vi "SeCrTs-DO Data FGV.vi"(0 "DO Values In":bool[](array[boolean]), 1 "Option":T1(ring)=enum."Start Pattern Mode", 5 "DO Channel Names":string[](array[string]), 7 "initiate":bool, 9 "Time Stamp In":timestamp, 11 "error in (no error)":errorcluster, 12 "DO Pattern Values In":bool[][](array[boolean])) -> (3 "Expected Completed Time (Pattern)":timestamp, 4 "DO Values Out":bool[](array[boolean]), 6 "All data out":waveform(dbl)[](array[waveform]), 8 "DO Channel Names Out":string[](array[string]), 10 "DO Waveform Out":digitalwaveform[](array[waveform]), 14 "Time Stamp Out":timestamp, 15 "error out":errorcluster)   [LabVIEW 2022 SP3]
uses:
  RT Controls/SeCrTs-FGV Read write.ctl
  <vilib>/Waveform/DTblOps.llb/DTbl Boolean Array to Digital.vi
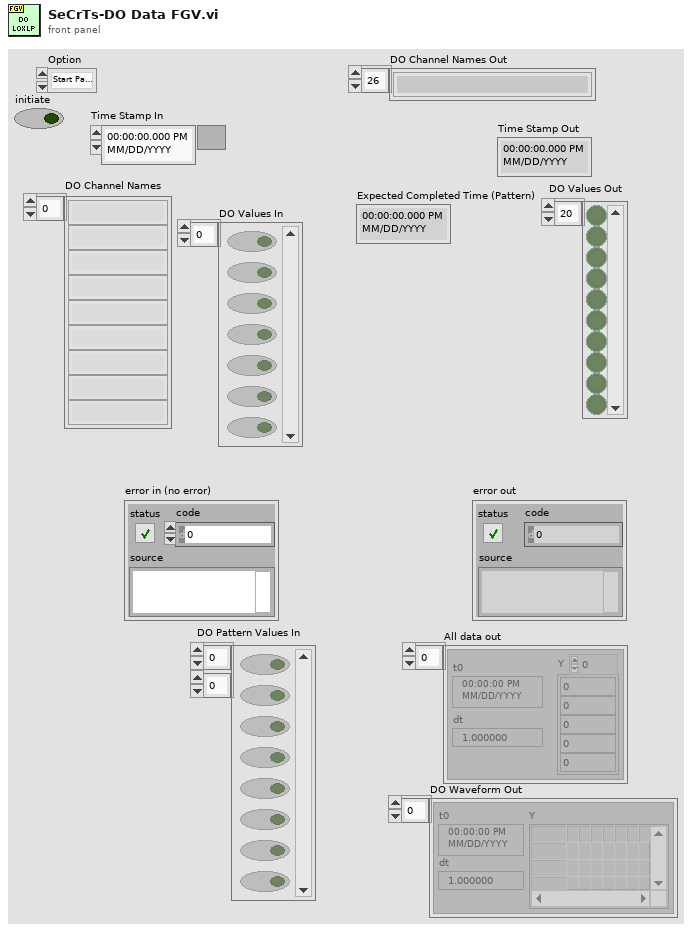
[diagram p1: front panel]
types:
  T1 = enum16{"Init", "Read", "Write 'All'", "Write 'n'", "Write Safe Value", "Write Start Time", "Overwrite Pattern", "Overwrite Pattern with Start", "Append Pattern", "Start Pattern Mode", "Abort Pattern Mode", "Read 1"}
  T2 = typedef "SeCrTs-FGV Read write.ctl" = enum16{"Write", "Read"}
  T3 = cluster{"Samples to Read":i32, "Pattern Mode?":bool, "dt(sec)":dbl, "DO Init Time (Samples)":i32, "dt per Read/Write":dbl, "Write Pointer":i32, "Pattern Size":i32, "Loop Rate (mSec)":i32, "Buffer Size (Samples)":i32, "Sampling rate":dbl, "Max DO Delay Time (samples)":dbl, "Min DO Delay Time (samples)":dbl, "Queue Size":i32, "DO Init Sample Duration (Sec)":dbl}
  T4 = cluster{"Pattern Size":i32, "Write Pointer":i32, "DO Channel Names":string[], "Pattern Mode?":bool, "DO Safe Waveform":waveform(dbl)[], "DO Safe Digital Waveform":digitalwaveform[], "DO Safe Values In":bool[], "dt per Read/Write":dbl}
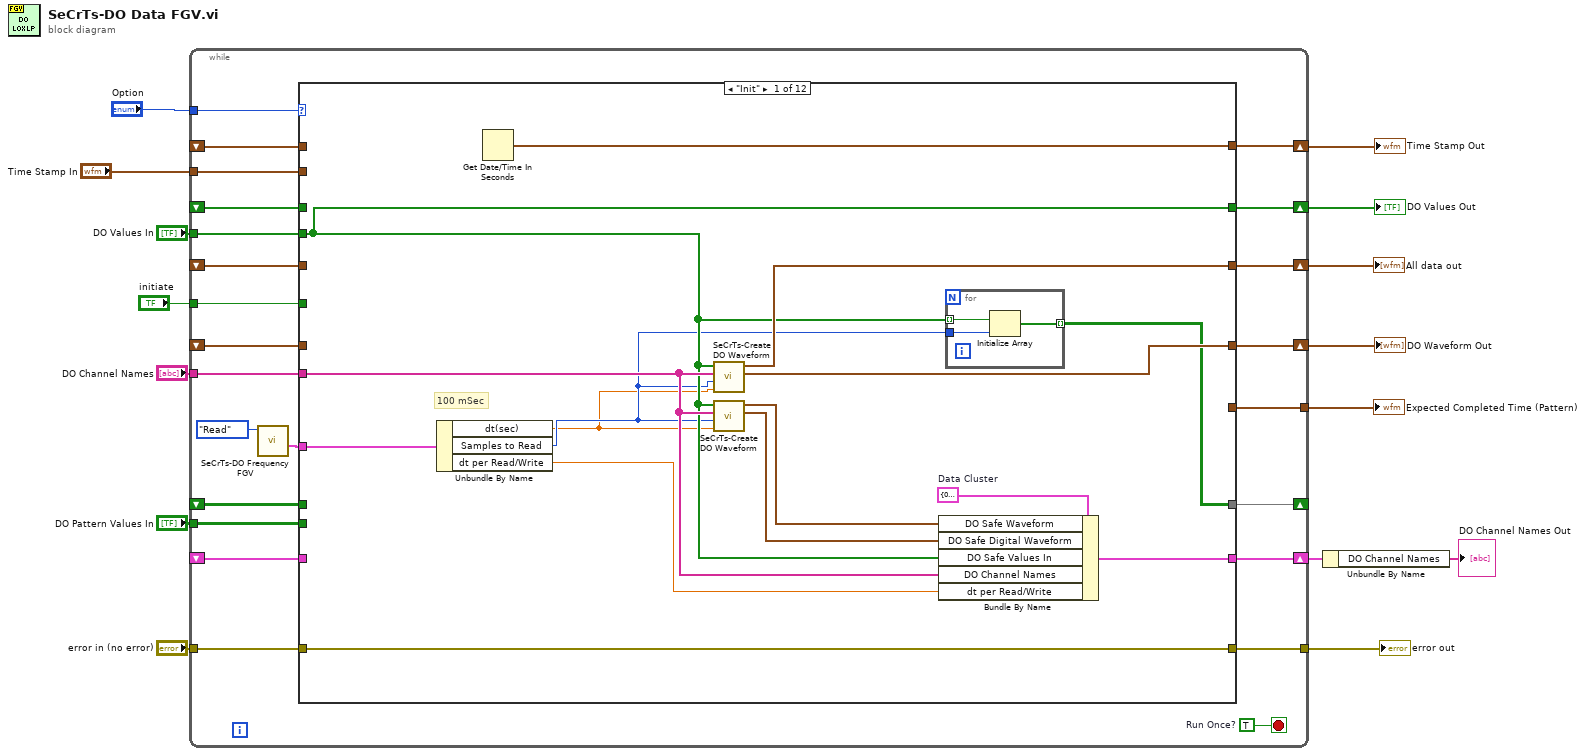
[diagram p0: block diagram]
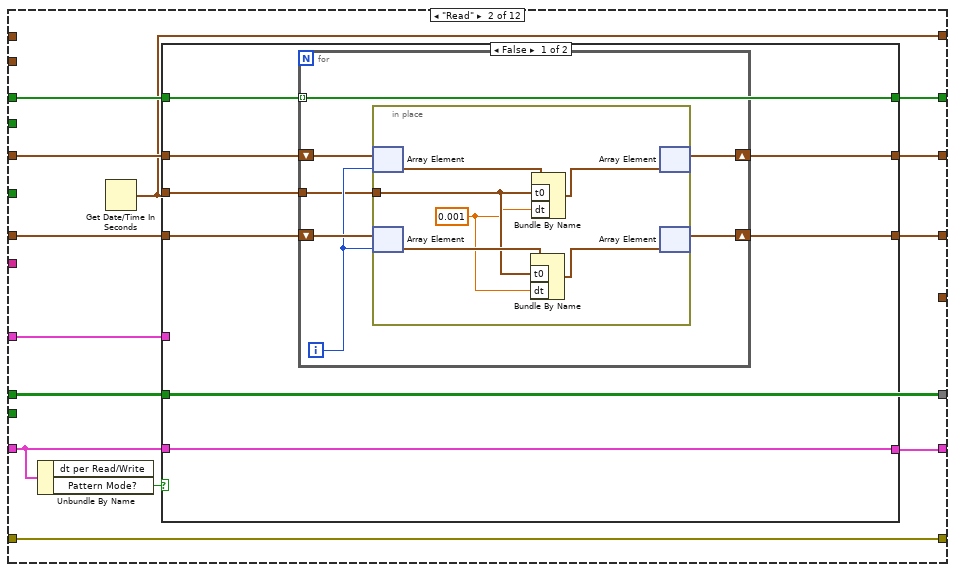
[diagram p2: hidden frame]
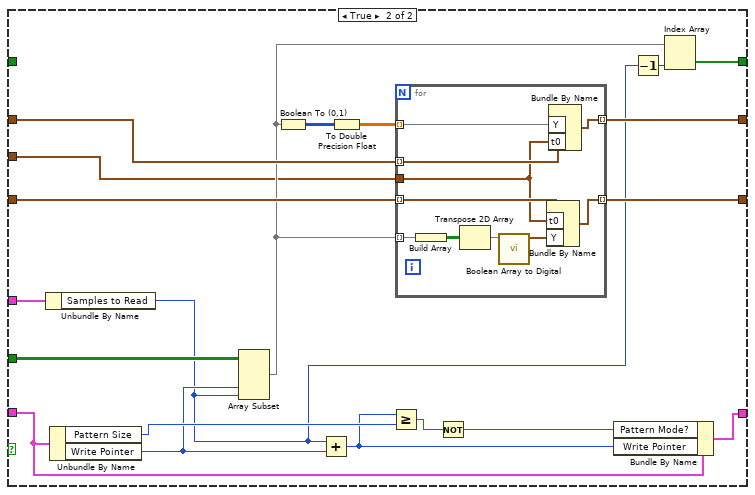
[diagram p3: hidden frame]
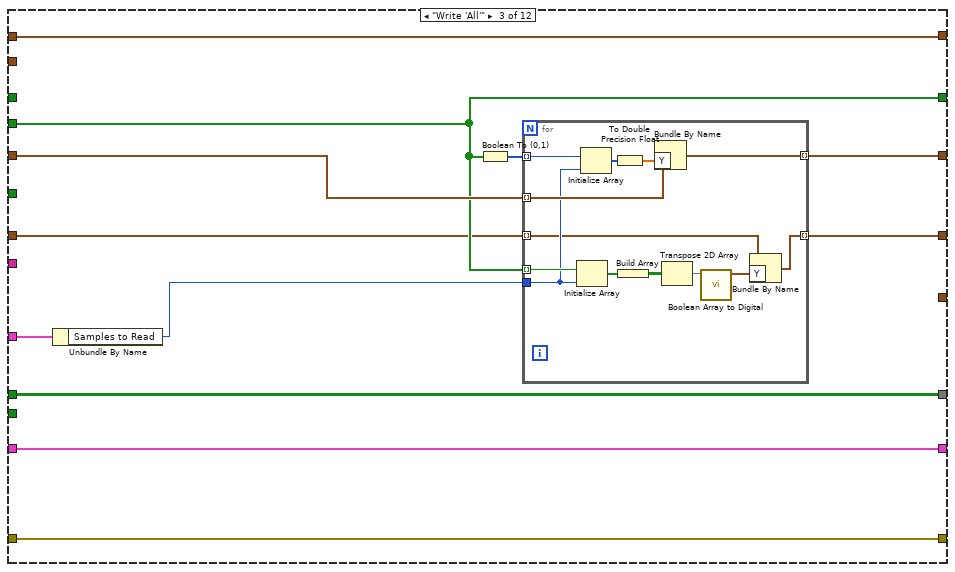
[diagram p4: hidden frame]
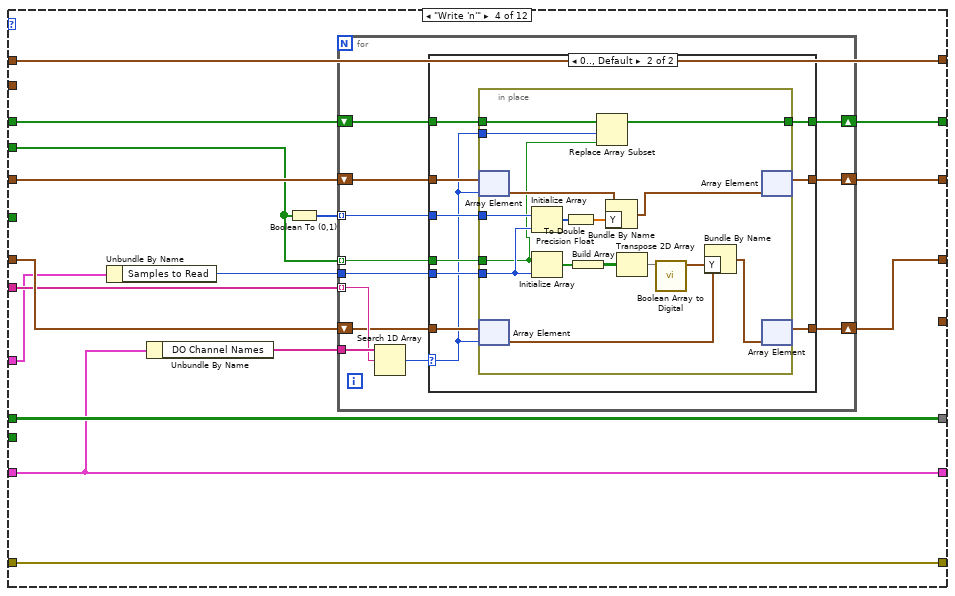
[diagram p5: hidden frame]
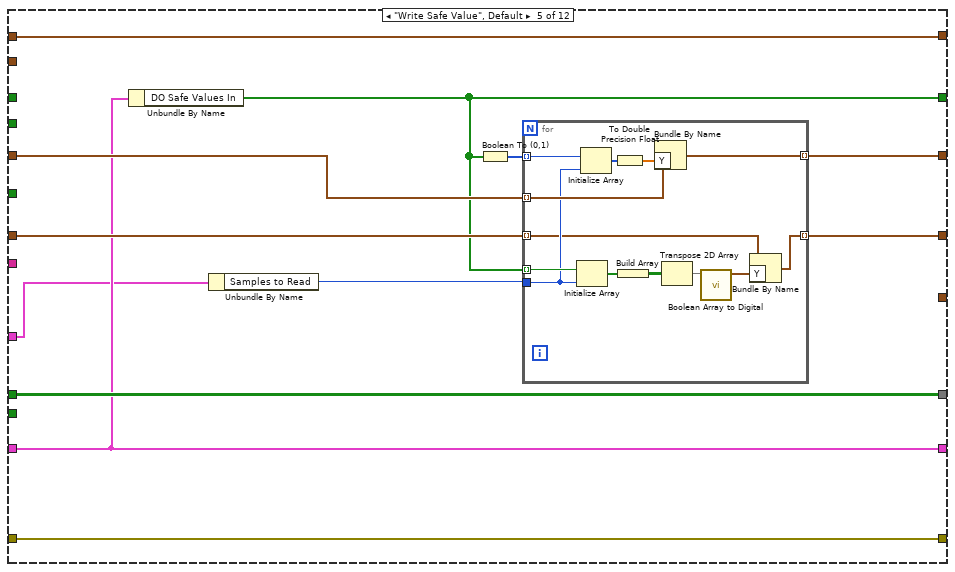
[diagram p7: hidden frame]
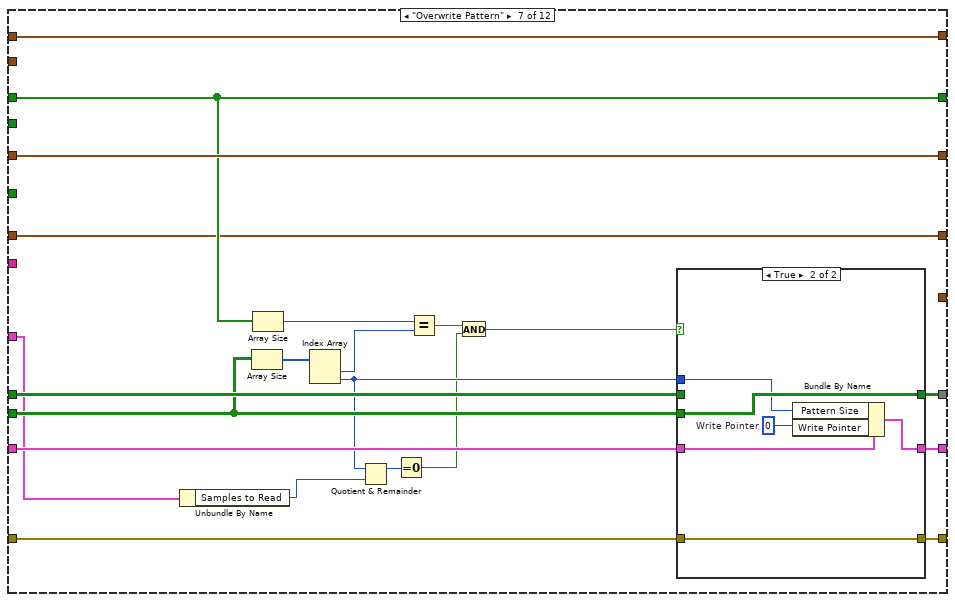
[diagram p9: hidden frame]
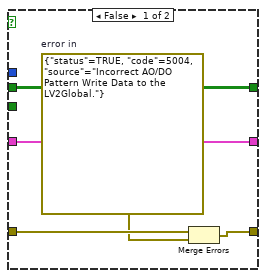
[diagram p10: hidden frame]
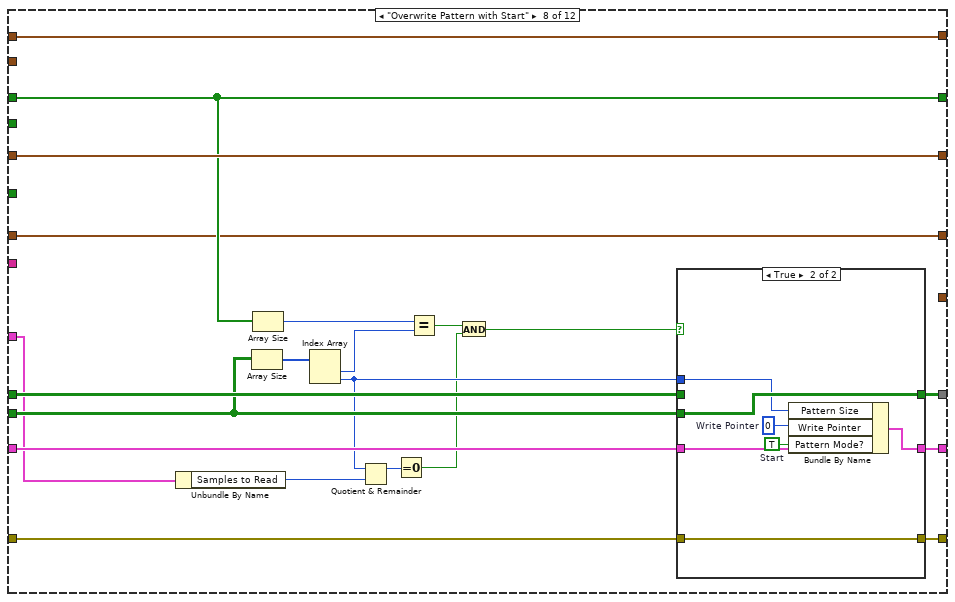
[diagram p11: hidden frame]
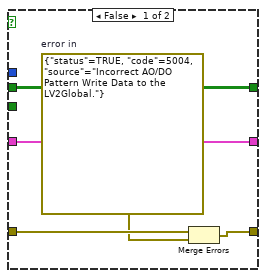
[diagram p12: hidden frame]
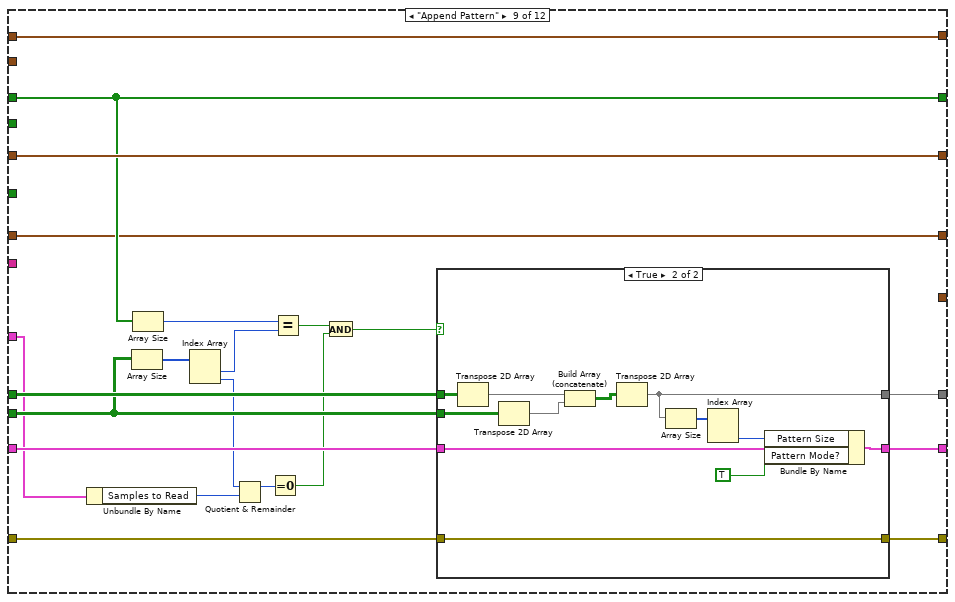
[diagram p13: hidden frame]
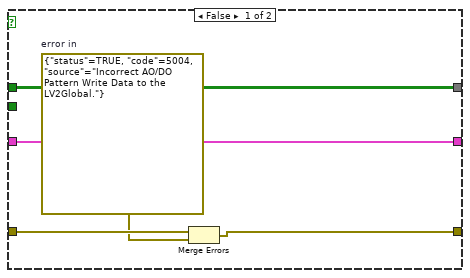
[diagram p14: hidden frame]
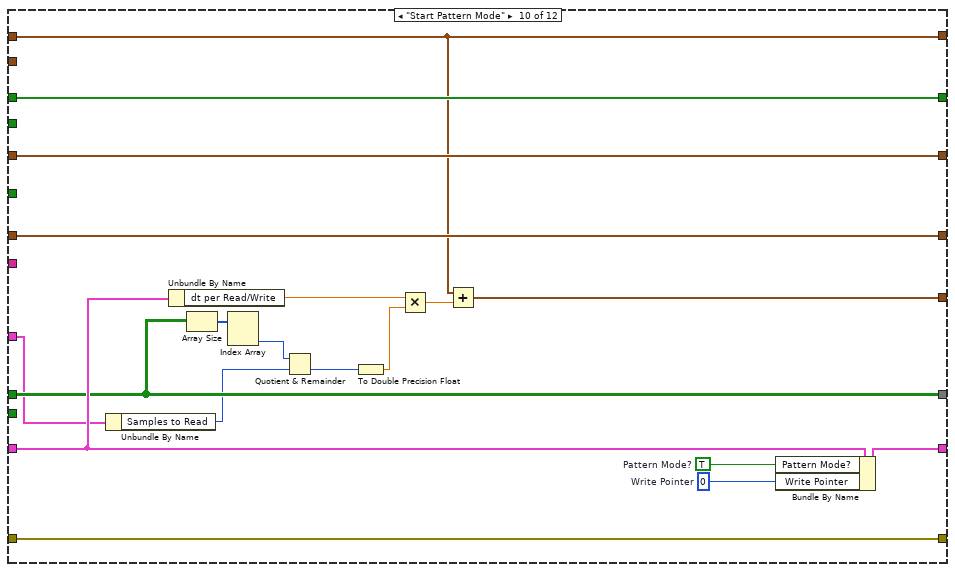
[diagram p15: hidden frame]
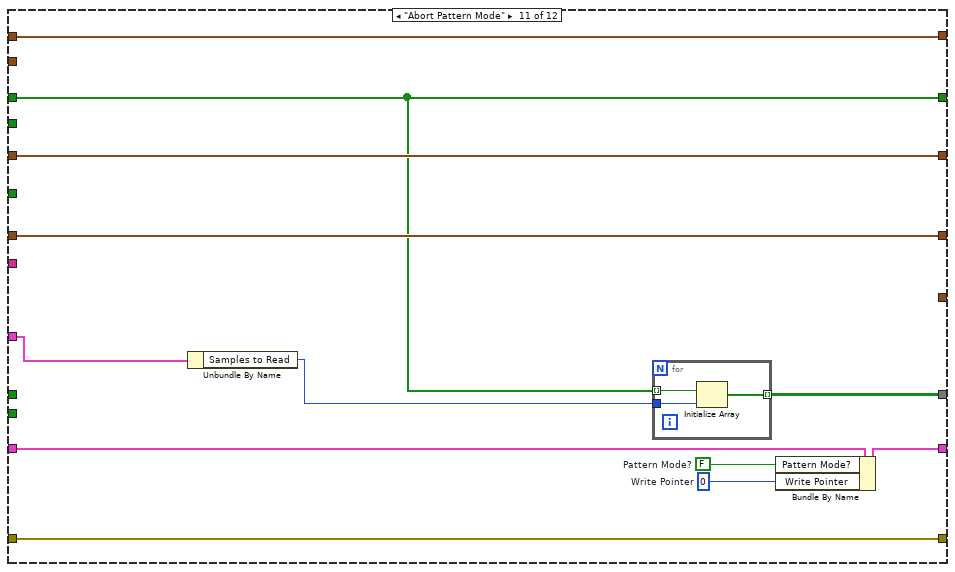
[diagram p16: hidden frame]
diagram:
  n1 = while {
    tunnel: "DO Values In" -> [w37]
    shift-right: [w38] -> w15
    shift-left: _ -> [w36]
    shift-right: [w35] -> w13
    shift-left: _ -> [w34]
    shift-right: [w33] -> w12
    shift-left: _ -> [w32]
    tunnel: "DO Pattern Values In" -> [w29]
    shift-right: [w30] -> _
    shift-left: _ -> [w28]
    shift-right: [w27] -> w3
    shift-left: _ -> [w26]
    tunnel: "error in (no error)" -> [w25]
    tunnel: [w24] -> w8
    tunnel: "DO Channel Names" -> [w23]
    shift-right: [w31] -> w11
    shift-left: _ -> [w22]
    tunnel: "Time Stamp In" -> [w21]
    tunnel: [w20] -> w5
    tunnel: "Option" -> [w19]
    tunnel: "initiate" -> [w17]
    stop <- w39 stop-if-true
    w39 = TRUE  # Run Once?
    n2 = call "SeCrTs-DO Frequency  FGV.vi"("Write/Read"=SeCrTs-FGV_Read_write."Read") -> ("DO Set Frequency (R)"=w18:T3)  [unwired: 9 in, 1 out]
    n3 = case shown="\"Init\"" w19 {
      tunnel: [w45 w61 w126 w147 w204 w233 w252 w284 w317 w355 w360 w377] -> w38
      tunnel: w37 -> [w45 _ w126 w156 _ _ _ _ _ _ _ _]
      tunnel: w36 -> [_ w66 _ w148 _ w233 w252 w284 w317 w355 w360 w377]
      tunnel: [w54 w58 w131 w160 w213 w227 w254 w286 w319 w347 w367 w371] -> w35
      tunnel: w34 -> [_ _ w131 w160 w213 _ w254 w286 w319 w347 w367 w371]
      tunnel: [w50 w62 w124 w154 w208 w232 w253 w285 w318 w354 w366 w372] -> w33
      tunnel: w32 -> [_ w67 w127 w157 w210 w232 w253 w285 w318 w354 w366 w372]
      tunnel: [w49 w63 w123 w153 w207 w231 w238 w270 w301 w353 w365 w373] -> w31
      tunnel: [w44 w60 w130 w159 w212 w230 w246 w278 w310 w346 w359 w376] -> w30
      tunnel: w29 -> [_ _ _ _ _ _ w244 w276 w308 _ _ _]
      tunnel: w28 -> [_ w60 w130 w159 w212 w230 w245 w277 w309 w346 _ w376]
      tunnel: [w51 w64 w129 w150 w205 w229 w247 w279 w312 w351 w362 w375] -> w27
      tunnel: w26 -> [_ w65 w129 w150 w205 w229 w248 w280 w313 w348 w364 w375]
      tunnel: w25 -> [w52 w70 w128 w158 w211 w228 w243 w275 w307 w352 w363 w374]
      tunnel: [w52 w70 w128 w158 w211 w228 w242 w274 w306 w352 w363 w374] -> w24
      tunnel: w23 -> [w48 _ _ w151 _ _ _ _ _ _ _ _]
      tunnel: w22 -> [_ w68 w122 w152 w206 w231 w238 w270 w301 w353 w365 w373]
      tunnel: w21 -> [_ _ _ _ _ w227 _ _ _ _ _ _]
      tunnel: [_ _ _ _ _ _ _ _ _ w340 _ _] -> w20
      tunnel: w18 -> [w43 w59 w121 w146 w202 _ w234 w266 w300 w337 w356 _]
      tunnel: w17 -> [_ _ _ _ _ _ _ _ _ _ _ _]
      frame "Init" {
        w53 = T4 {"Pattern Size"=0, "Write Pointer"=0, "DO Channel Names"=[], "Pattern Mode?"=FALSE, "DO Safe Waveform"=[], "DO Safe Digital Waveform"=[], "DO Safe Values In"=[], "dt per Read/Write"=100.0}  # Data Cluster
        # "100 mSec"
        n4 = Unbundle By Name(w43) -> ("dt(sec)"=w41:dbl, "Samples to Read"=w42:i32, "dt per Read/Write"=w40:dbl)
        n5 = Get Date/Time In Seconds() -> (seconds since 1Jan1904=w54:timestamp)
        n6 = call "SeCrTs-Create DO Waveform.vi"("dt(sec)"=w41, "Size"=w42, "DO Channel Names"=w48, "DO Values In"=w45) -> ("DO Digital Waveform"=w49:digitalwaveform[], "DO Waveform"=w50:waveform(dbl)[])  [unwired: 6 in]
        n7 = call "SeCrTs-Create DO Waveform.vi"("dt(sec)"=w41, "Size"=w42, "DO Channel Names"=w48, "DO Values In"=w45) -> ("DO Digital Waveform"=w46:digitalwaveform[], "DO Waveform"=w47:waveform(dbl)[])  [unwired: 6 in]
        n8 = Bundle By Name(cluster=w53, "DO Safe Waveform"=w47, "DO Safe Digital Waveform"=w46, "DO Safe Values In"=w45, "DO Channel Names"=w48, "dt per Read/Write"=w40) -> (w51:T4)
        n9 = for {
          tunnel: w42 -> [w57]
          tunnel: w45 -> [w56] mode=indexing
          tunnel: [w55] -> w44 mode=indexing
          n10 = Initialize Array(w56, w57) -> (w55:bool[])
        }
      }
      frame "Read" {
        n11 = Unbundle By Name(w65) -> ("Pattern Mode?"=w69:bool)  [unwired: 1 out]
        n12 = Get Date/Time In Seconds() -> (seconds since 1Jan1904=w58:timestamp)
        n13 = case shown="False" w69 {
          tunnel: w60 -> [_ w107]
          tunnel: w68 -> [w75 w106]
          tunnel: w67 -> [w76 w103]
          tunnel: w66 -> [w71 _]
          tunnel: w65 -> [w77 w109]
          tunnel: [w77 w108] -> w64
          tunnel: [w73 w105] -> w63
          tunnel: [w74 w104] -> w62
          tunnel: [w71 w101] -> w61
          tunnel: w58 -> [w72 w95]
          tunnel: w59 -> [_ w91]
          frame False {
            n14 = for {
              shift-right: [w80] -> w74
              shift-left: w76 -> [w83]
              shift-right: [w81] -> w73
              shift-left: w75 -> [w82]
              tunnel: w72 -> [w78]
              tunnel: w71 -> [_] mode=indexing
              i -> [w79]
              n15 = in-place {
                in-place-border: w78 -> [w85]
                w84 = 0.001 ("dt")
                n16 = in-place-array #1(w83, w79) -> (w89:waveform(dbl))
                n17 = in-place-array #2(w82, w79) -> (w87:digitalwaveform)
                n18 = Bundle By Name(cluster=w87, "t0"=w85, "dt"=w84) -> (w86:digitalwaveform)
                n19 = Bundle By Name(cluster=w89, "t0"=w85, "dt"=w84) -> (w88:waveform(dbl))
                n20 = in-place-array #1(w88) -> (w80:waveform(dbl)[])  [unwired: 1 out]
                n21 = in-place-array #2(w86) -> (w81:digitalwaveform[])  [unwired: 1 out]
              }
            }
          }
          frame True {
            n22 = Unbundle By Name(w91) -> ("Samples to Read"=w90:i32)
            n23 = Unbundle By Name(w109) -> ("Pattern Size"=w99:i32, "Write Pointer"=w94:i32)
            n24 = Array Subset(array=w107, index (col)=w94, length (col)=w90) -> (w102:bool[][])  [unwired: 2 in]
            n25 = Boolean To (0,1)(Boolean=w102) -> (0, 1=w97:i16[][])
            n26 = Add(x=w90, y=w94) -> (x+y=w93:i32)
            n27 = To Double Precision Float(number=w97) -> (double precision float=w96:dbl[][])
            n28 = Greater Or Equal?(x=w93, y=w99) -> (x >= y?=w98:bool)
            n29 = for {
              tunnel: [w119] -> w104 mode=indexing
              tunnel: w103 -> [w118] mode=indexing
              tunnel: w102 -> [w112] mode=indexing
              tunnel: [w115] -> w105 mode=indexing
              tunnel: w106 -> [w113] mode=indexing
              tunnel: w96 -> [w111] mode=indexing
              tunnel: w95 -> [w110]
              n30 = Build Array(w112) -> (w117:bool[][])
              n31 = Transpose 2D Array(2D array=w117) -> (transposed array=w114:bool[][])
              n32 = call-poly <vilib>:"Boolean Array to Digital.vi"("boolean array"=w114) -> ("digital data"=w116:digitaldata)  [unwired: 9 in, 1 out]
              n33 = Bundle By Name(cluster=w113, "t0"=w110, "Y"=w116) -> (w115:digitalwaveform)
              n34 = Bundle By Name(cluster=w118, "Y"=w111, "t0"=w110) -> (w119:waveform(dbl))
            }
            n35 = Not(x=w98) -> (.not. x?=w92:bool)
            n36 = Bundle By Name(cluster=w109, "Pattern Mode?"=w92, "Write Pointer"=w93) -> (w108:T4)
            n37 = Decrement(x=w90) -> (x-1=w100:i32)
            n38 = Index Array(array=w102, index (col)=w100) -> (element=w101:bool[])  [unwired: 1 in]
          }
        }
      }
      frame "Write 'All'" {
        n39 = Unbundle By Name(w121) -> ("Samples to Read"=w120:i32)
        n40 = Boolean To (0,1)(Boolean=w126) -> (0, 1=w125:i16[])
        n41 = for {
          tunnel: w125 -> [w143] mode=indexing
          tunnel: [w144] -> w124 mode=indexing
          tunnel: w120 -> [w138]
          tunnel: w127 -> [w140] mode=indexing
          tunnel: w126 -> [w139] mode=indexing
          tunnel: [w134] -> w123 mode=indexing
          tunnel: w122 -> [w132] mode=indexing
          n42 = Initialize Array(w139, w138) -> (w137:bool[])
          n43 = Initialize Array(w143, w138) -> (w142:i16[])
          n44 = To Double Precision Float(number=w142) -> (double precision float=w141:dbl[])
          n45 = Build Array(w137) -> (w136:bool[][])
          n46 = Bundle By Name(cluster=w140, "Y"=w141) -> (w144:waveform(dbl))
          n47 = Transpose 2D Array(2D array=w136) -> (transposed array=w133:bool[][])
          n48 = call-poly <vilib>:"Boolean Array to Digital.vi"("boolean array"=w133) -> ("digital data"=w135:digitaldata)  [unwired: 9 in, 1 out]
          n49 = Bundle By Name(cluster=w132, "Y"=w135) -> (w134:digitalwaveform)
        }
      }
      frame "Write 'n'" {
        n50 = Unbundle By Name(w146) -> ("Samples to Read"=w145:i32)
        n51 = Unbundle By Name(w150) -> ("DO Channel Names"=w149:string[])
        n52 = Boolean To (0,1)(Boolean=w156) -> (0, 1=w155:i16[])
        n53 = for {
          tunnel: w155 -> [w171] mode=indexing
          tunnel: w145 -> [w169]
          tunnel: w156 -> [w170] mode=indexing
          shift-right: [w163] -> w153
          shift-left: w152 -> [w165]
          tunnel: w151 -> [w167] mode=indexing
          tunnel: w149 -> [w168]
          shift-right: [w172] -> w154
          shift-left: w157 -> [w164]
          shift-right: [w161] -> w147
          shift-left: w148 -> [w162]
          n54 = Search 1D Array(1D array=w168, element=w167) -> (index of element=w166:i32)  [unwired: 1 in]
          n55 = case shown="0.., Default" w166 {
            selector: w166 -> [_ w176]
            tunnel: [w175 w180] -> w172
            tunnel: w171 -> [_ w185]
            tunnel: w170 -> [_ w184]
            tunnel: w169 -> [_ w183]
            tunnel: w165 -> [w174 w182]
            tunnel: w164 -> [w175 w181]
            tunnel: [w174 w179] -> w163
            tunnel: w162 -> [w173 w178]
            tunnel: [w173 w177] -> w161
            frame -1 {
            }
            frame 0.., Default {
              n56 = in-place {
                in-place-border: w185 -> [w201]
                in-place-border: w184 -> [w186]
                in-place-border: w183 -> [w198]
                in-place-border: w178 -> [w189]
                in-place-border: [w188] -> w177
                in-place-border: w176 -> [w187]
                n57 = in-place-array #3(w181, w176) -> (w191:waveform(dbl))
                n58 = in-place-array #4(w182, w176) -> (w193:digitalwaveform)
                n59 = Initialize Array(w201, w198) -> (w200:i16[])
                n60 = Initialize Array(w186, w198) -> (w197:bool[])
                n61 = To Double Precision Float(number=w200) -> (double precision float=w199:dbl[])
                n62 = Build Array(w197) -> (w196:bool[][])
                n63 = Replace Array Subset(array=w189, new element=w186, index=w187) -> (w188:bool[])
                n64 = Bundle By Name(cluster=w191, "Y"=w199) -> (w192:waveform(dbl))
                n65 = Transpose 2D Array(2D array=w196) -> (transposed array=w194:bool[][])
                n66 = call-poly <vilib>:"Boolean Array to Digital.vi"("boolean array"=w194) -> ("digital data"=w195:digitaldata)  [unwired: 9 in, 1 out]
                n67 = Bundle By Name(cluster=w193, "Y"=w195) -> (w190:digitalwaveform)
                n68 = in-place-array #3(w192) -> (w180:waveform(dbl)[])  [unwired: 1 out]
                n69 = in-place-array #4(w190) -> (w179:digitalwaveform[])  [unwired: 1 out]
              }
            }
          }
        }
      }
      frame "Write Safe Value", Default {
        n70 = Unbundle By Name(w205) -> ("DO Safe Values In"=w204:bool[])
        n71 = Unbundle By Name(w202) -> ("Samples to Read"=w203:i32)
        n72 = Boolean To (0,1)(Boolean=w204) -> (0, 1=w209:i16[])
        n73 = for {
          tunnel: w209 -> [w225] mode=indexing
          tunnel: [w226] -> w208 mode=indexing
          tunnel: w203 -> [w220]
          tunnel: w210 -> [w222] mode=indexing
          tunnel: w204 -> [w221] mode=indexing
          tunnel: [w216] -> w207 mode=indexing
          tunnel: w206 -> [w214] mode=indexing
          n74 = Initialize Array(w221, w220) -> (w219:bool[])
          n75 = Initialize Array(w225, w220) -> (w224:i16[])
          n76 = To Double Precision Float(number=w224) -> (double precision float=w223:dbl[])
          n77 = Build Array(w219) -> (w218:bool[][])
          n78 = Bundle By Name(cluster=w222, "Y"=w223) -> (w226:waveform(dbl))
          n79 = Transpose 2D Array(2D array=w218) -> (transposed array=w215:bool[][])
          n80 = call-poly <vilib>:"Boolean Array to Digital.vi"("boolean array"=w215) -> ("digital data"=w217:digitaldata)  [unwired: 9 in, 1 out]
          n81 = Bundle By Name(cluster=w214, "Y"=w217) -> (w216:digitalwaveform)
        }
      }
      frame "Write Start Time" {
      }
      frame "Overwrite Pattern" {
        n82 = Unbundle By Name(w234) -> ("Samples to Read"=w235:i32)
        n83 = Array Size(array=w244) -> (size(s)=w251:i32[])
        n84 = Array Size(array=w252) -> (size(s)=w249:i32)
        n85 = Index Array(array=w251) -> (element #1=w250:i32, element #2=w241:i32)  [unwired: 2 in]
        n86 = Quotient & Remainder(x=w241, y=w235) -> (x-y*floor(x/y)=w240:i32)  [unwired: 1 out]
        n87 = Equal To 0?(x=w240) -> (x = 0?=w236:bool)
        n88 = Equal?(x=w249, y=w250) -> (x = y?=w237:bool)
        n89 = And(x=w237, y=w236) -> (x .and. y?=w239:bool)
        n90 = case shown="True" w239 {
          tunnel: w248 -> [w259 w265]
          tunnel: [w259 w264] -> w247
          tunnel: w241 -> [_ w260]
          tunnel: [w258 w262] -> w246
          tunnel: w245 -> [w258 _]
          tunnel: w244 -> [_ w262]
          tunnel: w243 -> [w257 w261]
          tunnel: [w256 w261] -> w242
          frame False {
            w255 = errorcluster {"status"=TRUE, "code"=5004, "source"="Incorrect AO/DO Pattern Write Data to the LV2Global."}  # error in
            n91 = Merge Errors(w257, w255) -> (w256:errorcluster)
          }
          frame True {
            w263 = 0  # Write Pointer
            n92 = Bundle By Name(cluster=w265, "Pattern Size"=w260, "Write Pointer"=w263) -> (w264:T4)
          }
        }
      }
      frame "Overwrite Pattern with Start" {
        n93 = Unbundle By Name(w266) -> ("Samples to Read"=w267:i32)
        n94 = Array Size(array=w276) -> (size(s)=w283:i32[])
        n95 = Array Size(array=w284) -> (size(s)=w281:i32)
        n96 = Index Array(array=w283) -> (element #1=w282:i32, element #2=w273:i32)  [unwired: 2 in]
        n97 = Quotient & Remainder(x=w273, y=w267) -> (x-y*floor(x/y)=w272:i32)  [unwired: 1 out]
        n98 = Equal To 0?(x=w272) -> (x = 0?=w268:bool)
        n99 = Equal?(x=w281, y=w282) -> (x = y?=w269:bool)
        n100 = And(x=w269, y=w268) -> (x .and. y?=w271:bool)
        n101 = case shown="True" w271 {
          tunnel: w280 -> [w291 w298]
          tunnel: [w291 w297] -> w279
          tunnel: w273 -> [_ w292]
          tunnel: [w290 w295] -> w278
          tunnel: w277 -> [w290 _]
          tunnel: w276 -> [_ w295]
          tunnel: w275 -> [w289 w294]
          tunnel: [w288 w294] -> w274
          frame False {
            w287 = errorcluster {"status"=TRUE, "code"=5004, "source"="Incorrect AO/DO Pattern Write Data to the LV2Global."}  # error in
            n102 = Merge Errors(w289, w287) -> (w288:errorcluster)
          }
          frame True {
            w293 = TRUE  # Start
            w296 = 0  # Write Pointer
            n103 = Bundle By Name(cluster=w298, "Pattern Size"=w292, "Write Pointer"=w296, "Pattern Mode?"=w293) -> (w297:T4)
          }
        }
      }
      frame "Append Pattern" {
        n104 = Unbundle By Name(w300) -> ("Samples to Read"=w299:i32)
        n105 = Array Size(array=w308) -> (size(s)=w316:i32[])
        n106 = Array Size(array=w317) -> (size(s)=w314:i32)
        n107 = Index Array(array=w316) -> (element #1=w315:i32, element #2=w304:i32)  [unwired: 2 in]
        n108 = Quotient & Remainder(x=w304, y=w299) -> (x-y*floor(x/y)=w305:i32)  [unwired: 1 out]
        n109 = Equal To 0?(x=w305) -> (x = 0?=w302:bool)
        n110 = Equal?(x=w314, y=w315) -> (x = y?=w311:bool)
        n111 = And(x=w311, y=w302) -> (x .and. y?=w303:bool)
        n112 = case shown="True" w303 {
          tunnel: w313 -> [w324 w336]
          tunnel: [w324 w335] -> w312
          tunnel: [w323 w327] -> w310
          tunnel: w309 -> [w323 w333]
          tunnel: w308 -> [_ w332]
          tunnel: w307 -> [w322 w334]
          tunnel: [w321 w334] -> w306
          frame False {
            w320 = errorcluster {"status"=TRUE, "code"=5004, "source"="Incorrect AO/DO Pattern Write Data to the LV2Global."}  # error in
            n113 = Merge Errors(w322, w320) -> (w321:errorcluster)
          }
          frame True {
            n114 = Transpose 2D Array(2D array=w333) -> (transposed array=w331:bool[][])
            n115 = Transpose 2D Array(2D array=w332) -> (transposed array=w330:bool[][])
            n116 = Build Array (concatenate)(w331, w330) -> (w329:bool[][])
            n117 = Transpose 2D Array(2D array=w329) -> (transposed array=w327:bool[][])
            n118 = Array Size(array=w327) -> (size(s)=w328:i32[])
            n119 = Index Array(array=w328) -> (element #2=w325:i32)  [unwired: 2 in, 1 out]
            n120 = Bundle By Name(cluster=w336, "Pattern Size"=w325, "Pattern Mode?"=TRUE) -> (w335:T4)
          }
        }
      }
      frame "Start Pattern Mode" {
        w349 = 0  # Write Pointer
        w350 = TRUE  # Pattern Mode?
        n121 = Unbundle By Name(w337) -> ("Samples to Read"=w338:i32)
        n122 = Unbundle By Name(w348) -> ("dt per Read/Write"=w343:dbl)
        n123 = Array Size(array=w346) -> (size(s)=w345:i32[])
        n124 = Index Array(array=w345) -> (element #2=w344:i32)  [unwired: 2 in, 1 out]
        n125 = Quotient & Remainder(x=w344, y=w338) -> (floor(x/y)=w339:i32)  [unwired: 1 out]
        n126 = To Double Precision Float(number=w339) -> (double precision float=w341:dbl)
        n127 = Multiply(x=w343, y=w341) -> (x*y=w342:dbl)
        n128 = Add(x=w347, y=w342) -> (x+y=w340:timestamp)
        n129 = Bundle By Name(cluster=w348, "Pattern Mode?"=w350, "Write Pointer"=w349) -> (w351:T4)
      }
      frame "Abort Pattern Mode" {
        w361 = 0  # Write Pointer
        w358 = FALSE  # Pattern Mode?
        n130 = Unbundle By Name(w356) -> ("Samples to Read"=w357:i32)
        n131 = for {
          tunnel: w357 -> [w370]
          tunnel: w360 -> [w369] mode=indexing
          tunnel: [w368] -> w359 mode=indexing
          n132 = Initialize Array(w369, w370) -> (w368:bool[])
        }
        n133 = Bundle By Name(cluster=w364, "Pattern Mode?"=w358, "Write Pointer"=w361) -> (w362:T4)
      }
      frame "Read 1" {
      }
    }
  }
  "error out" <- w8
  "DO Values Out" <- w15
  "Time Stamp Out" <- w13
  "All data out" <- w12
  "DO Waveform Out" <- w11
  "Expected Completed Time (Pattern)" <- w5
  n134 = Unbundle By Name(w3) -> ("DO Channel Names"=→"DO Channel Names Out":string[])
